vi "Check for Weighting Conflict.vi"(0 "weighting filter":T1(ring), 1 "channel info":T2={"sensor sensitivity [mV/EU]"=1000.0, "engineering units"=1, "dB reference [EU]"=1.0, "custom label"="EU", "weighting filter"=0, "pregain [dB]"=0.0} {"pregain [dB]" format="%.2f"; "weighting filter" items=["Linear", "A-weighting", "B-weighting", "C-weighting", "ITU-R 468-4", "Dolby", "CCITT", "C-message"]; "dB reference [EU]" format="%^.1e"; "engineering units" items=["custom..."=0, "V"=1, "A"=21, "Pa"=2, "N"=20, "g"=3, "m/s^2"=4, "m/s"=5, "m"=6, "mm/s"=12, "mm"=13, "microns/s"=14, "microns"=15, "in/s^2"=7, "in/s"=8, "in"=9, "mils/s"=10, "mils"=11, "rad/s^2"=16, "rad/s"=17, "rad"=18, "strain"=19]; "sensor sensitivity [mV/EU]" format="%.2f"}) -> (2 "weighting to apply":T1(ring), 3 "weighting units":T1(ring), 4 "weighting conflict":bool)   [LabVIEW 2017]
uses:
  <vilib>/addons/Sound and Vibration/compatibility/Controls/svl_Channel Info.ctl
  <vilib>/addons/Sound and Vibration/compatibility/Controls/svl_Engineering Units Text Ring.ctl
  <vilib>/addons/Sound and Vibration/compatibility/Controls/svl_Weighting Filter Text Ring.ctl
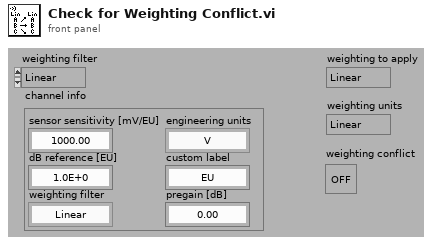
[diagram p1: front panel]
types:
  T1 = enum16{"Linear", "A-weighting", "B-weighting", "C-weighting"}
  T2 = typedef "svl_Channel Info.ctl" = cluster{"sensor sensitivity [mV/EU]":dbl, "engineering units":T3, "dB reference [EU]":dbl, "custom label":string, "weighting filter":T4, "pregain [dB]":dbl}
  T3 = typedef "svl_Engineering Units Text Ring.ctl" = u16
  T4 = typedef "svl_Weighting Filter Text Ring.ctl" = u16
  T5 = typedef "svc_Weighting Filter Text Ring.ctl" = u16
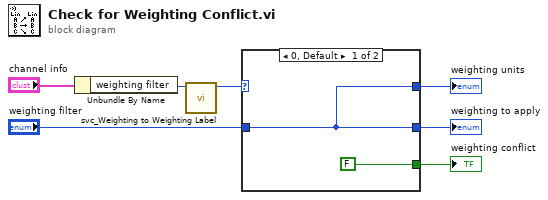
[diagram p0: block diagram]
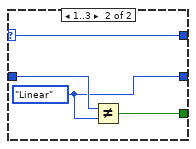
[diagram p2: hidden frame]
diagram:
  n1 = Unbundle By Name("channel info") -> ("weighting filter"=w2:T4)
  n2 = call <vilib>:"svc_Weighting to Weighting Label.vi"("weighting filter"=w2) -> ("weighting enum"=w1:T5)  [unwired: 9 in, 1 out]
  n3 = case shown="0, Default" w1 {
    selector: w1 -> [_ w10]
    tunnel: "weighting filter" -> [w8 w13]
    tunnel: [w8 w11] -> w5
    tunnel: [FALSE w12] -> w4
    tunnel: [w8 w10] -> w3
    frame 0, Default {
    }
    frame 1..3 {
      w11 = T1."Linear" ("y")
      n4 = Not Equal?(x=w13, y=w11) -> (x != y?=w12:bool)
    }
  }
  "weighting to apply" <- w5
  "weighting conflict" <- w4
  "weighting units" <- w3
